vi "DataPacker_SetupSSH.vi"(0 "DataPacker in":refnum<class "DataPacker.lvclass">, 1 "ssh hostname":string, 2 "ssh host port":i32, 3 "username":string, 4 "password":string, 5 "error in (no error)":errorcluster) -> (14 "DataPacker out":refnum<class "DataPacker.lvclass">, 19 "error out":errorcluster)   [LabVIEW 2018, in "DataPacker.lvclass"]
uses:
  DataPacker.lvclass
  DataPacker.lvclass/DataPacker.ctl
  Utilities/SSH_TUNNEL.lvclass/SSH_TUNNEL.ctl
  Utilities/SSH_TUNNEL.lvclass
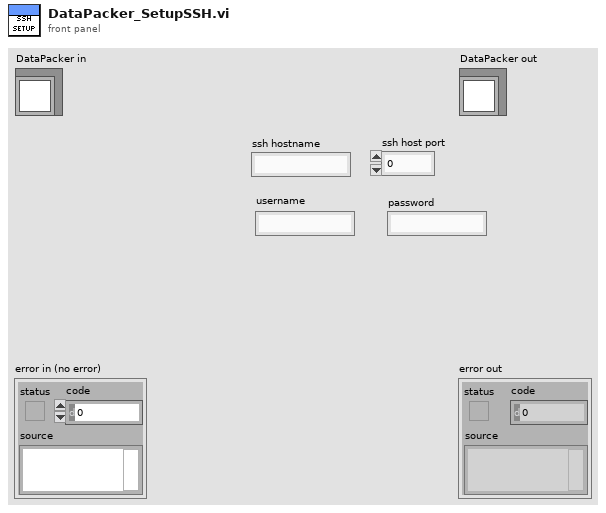
[diagram p1: front panel]
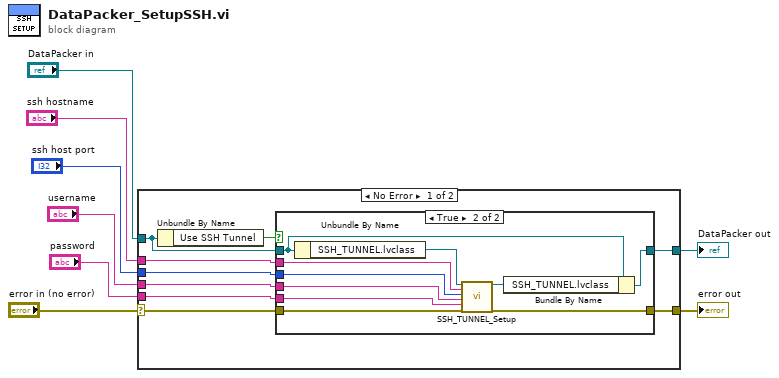
[diagram p0: block diagram]
diagram:
  n1 = case shown="No Error" "error in (no error)" {
    selector: "error in (no error)" -> [w12 w31]
    tunnel: [w11 w31] -> w7
    tunnel: [w9 w30] -> w5
    tunnel: "DataPacker in" -> [w10 w30]
    tunnel: "password" -> [w16 _]
    tunnel: "ssh hostname" -> [w15 _]
    tunnel: "ssh host port" -> [w14 _]
    tunnel: "username" -> [w13 _]
    frame No Error {
      n2 = Unbundle By Name(w10) -> ("Use SSH Tunnel"=w17:bool)
      n3 = case shown="True" w17 {
        tunnel: w16 -> [_ w29]
        tunnel: w15 -> [_ w28]
        tunnel: w14 -> [_ w27]
        tunnel: w13 -> [_ w26]
        tunnel: w12 -> [w18 w25]
        tunnel: [w18 w24] -> w11
        tunnel: w10 -> [w19 w20]
        tunnel: [w19 w21] -> w9
        frame False {
        }
        frame True {
          n4 = Unbundle By Name(w20) -> ("SSH_TUNNEL.lvclass"=w22:refnum<class "SSH_TUNNEL.lvclass">)
          n5 = call "SSH_TUNNEL_Setup.vi"("SSH_TUNNEL in"=w22, "ssh hostname"=w28, "ssh host port"=w27, "username"=w26, "password"=w29, "error in (no error)"=w25) -> ("SSH_TUNNEL out"=w23:refnum<class "SSH_TUNNEL.lvclass">, "error out"=w24:errorcluster)  [unwired: 12 in]
          n6 = Bundle By Name(cluster=w20, "SSH_TUNNEL.lvclass"=w23) -> (w21:refnum<class "DataPacker.lvclass">)
        }
      }
    }
    frame Error {
    }
  }
  "error out" <- w7
  "DataPacker out" <- w5
